vi "_CH375_Open.vi"(8 "Error In":errorcluster caption="错误输入", 11 "USB状态":bool) -> (0 "Error Out":errorcluster caption="错误输出", 3 "设备连接状况":bool)   [LabVIEW 2020, in "CH375.lvlib"]
uses:
  CH375.lvlib
  CH375DLL64.dll
panel:
  in  "衰减模式电压（V）":dbl(slide)=1.0303030303030305 scale=0.0..2.0
  in  "电机驱动电流（未标定）":dbl(slide)=1.5 scale=0.0..2.0
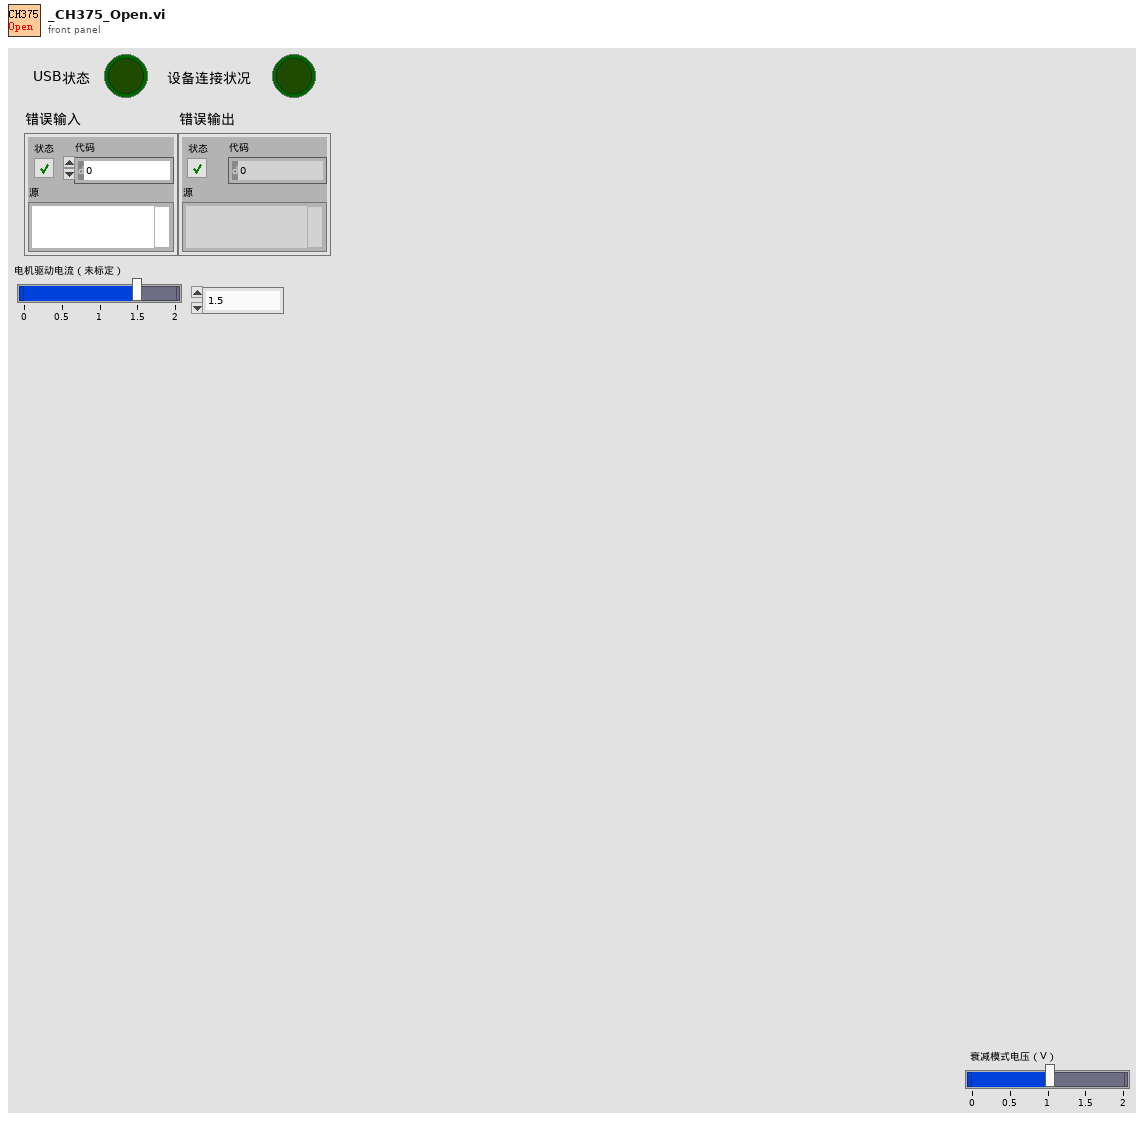
[diagram p1: front panel]
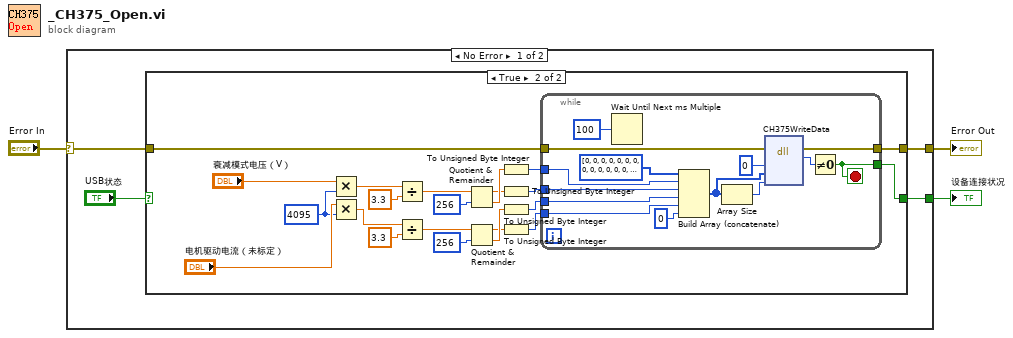
[diagram p0: block diagram]
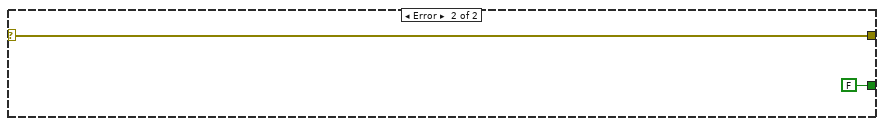
[diagram p3: hidden frame]
diagram:
  n1 = case shown="No Error" "Error In" {
    selector: "Error In" -> [w4 w47]
    tunnel: [w7 w47] -> w2
    tunnel: [w6 FALSE] -> w1
    frame No Error {
      n2 = case shown="True" "USB状态" {
        selector: "USB状态" -> [w8 _]
        tunnel: [w9 w12] -> w7
        tunnel: w4 -> [w9 w11]
        tunnel: [w8 w10] -> w6
        frame False {
        }
        frame True {
          w17 = u16 4095 ("y")
          n3 = Multiply(x="衰减模式电压（V）", y=w17) -> (x*y=w18:dbl)
          n4 = Multiply(x="电机驱动电流（未标定）", y=w17) -> (x*y=w24:dbl)
          n5 = Divide(x=w18, y=3.3) -> (x/y=w19:dbl)
          n6 = Divide(x=w24, y=3.3) -> (x/y=w25:dbl)
          n7 = Quotient & Remainder(x=w19, y=u16 256) -> (x-y*floor(x/y)=w20:dbl, floor(x/y)=w21:dbl)
          n8 = Quotient & Remainder(x=w25, y=u16 256) -> (x-y*floor(x/y)=w26:dbl, floor(x/y)=w27:dbl)
          n9 = To Unsigned Byte Integer(number=w21) -> (unsigned 8bit integer=w22:u8)
          n10 = To Unsigned Byte Integer(number=w20) -> (unsigned 8bit integer=w23:u8)
          n11 = To Unsigned Byte Integer(number=w27) -> (unsigned 8bit integer=w28:u8)
          n12 = To Unsigned Byte Integer(number=w26) -> (unsigned 8bit integer=w29:u8)
          n13 = while {
            tunnel: w11 -> [w45]
            tunnel: [w44] -> w12
            tunnel: w22 -> [w37]
            tunnel: w23 -> [w36]
            tunnel: w28 -> [w35]
            tunnel: w29 -> [w34]
            tunnel: [w32] -> w10
            stop <- w32 stop-if-true
            n14 = Wait Until Next ms Multiple(millisecond multiple=u32 100 ("毫秒倍数")) -> ()  [unwired: 1 out]
            n15 = Build Array (concatenate)(i32[] [0, 0, 0, 0, 0, 0, 0, 0, 0, 0, 0, 0, 0, 0, 0, 0, 0, 0, 0, 0, 0, 0, 0, 0, 0, 0, 0, 0, 0, 0, 0, 0, 0, 0, 85] ("添加的数组"), w37, w36, w35, w34, 0 ("元素")) -> (w39:i32[])
            n16 = Array Size(array=w39) -> (size(s)=w42:i32)
            n17 = dll-call lib="D:/Project NJU/lib/CH375/CH375DLL64.dll" fn="CH375WriteData"(error in=w45, "iIndex"=u8 0, "oBuffer"=w39, "ioLength"=w42) -> (error out=w44:errorcluster, "返回类型"=w40:i32)  [unwired: 3 in, 3 out]
            n18 = Not Equal To 0?(x=w40) -> (x != 0?=w32:bool)
          }
        }
      }
    }
    frame Error {
    }
  }
  "Error Out" <- w2
  "设备连接状况" <- w1
